vi "Single Channel Strain Configure 4Wire.vi"(5 "Channel":string, 6 "SampTime":dbl, 7 "SampCount":i32 format="%.0g", 8 "error in (no error)":errorcluster {"code" format="%.0x"}, 9 "GaugeFactor":dbl, 10 "GaugeResistance":dbl, 11 "instrument handle":refnum<k15>) -> (0 "error out":errorcluster {"code" format="%.0x"}, 3 "instrument handle out":refnum<k15>)   [LabVIEW 2020, in "Keysight DAQ970.lvlib"]
doc: "Configures a single channel for direct 4-wire strain gauge DMM digitizing, but they do not initiate the digitizing. This command redefines the scan list."
uses:
  Keysight DAQ970.lvlib
  KtDAQ970.dll
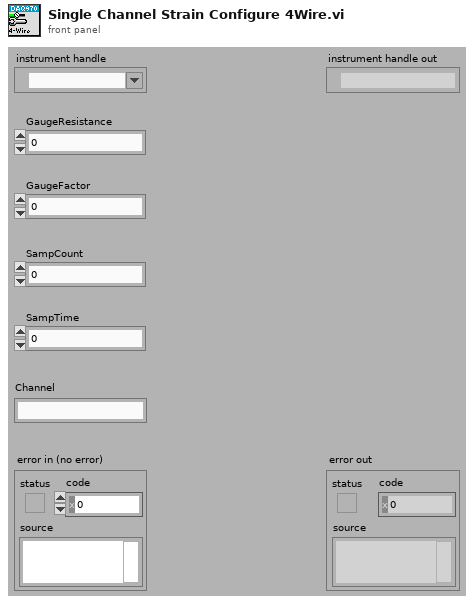
[diagram p1: front panel]
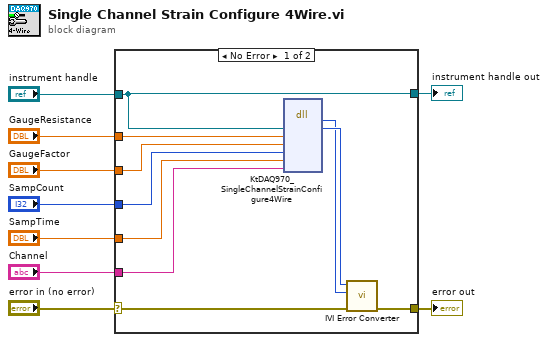
[diagram p0: block diagram]
diagram:
  n1 = case shown="No Error" "error in (no error)" {
    selector: "error in (no error)" -> [w10 w21]
    tunnel: [w17 w21] -> w9
    tunnel: "instrument handle" -> [w11 w20]
    tunnel: "GaugeResistance" -> [w16 _]
    tunnel: "GaugeFactor" -> [w15 _]
    tunnel: "SampCount" -> [w14 _]
    tunnel: "SampTime" -> [w13 _]
    tunnel: "Channel" -> [w12 _]
    tunnel: [w11 w20] -> w1
    frame No Error {
      n2 = dll-call lib="KtDAQ970**.dll" fn="KtDAQ970_SingleChannelStrainConfigure4Wire"("Vi"=w11, "GaugeResistance"=w16, "GaugeFactor"=w15, "SampCount"=w14, "SampTime"=w13, "Channel"=w12) -> (w18:i32, "Vi"=w19:u32)  [unwired: 8 in, 2 out]
      n3 = call "IVI Error Converter.vi"("error in (no error)"=w10, "IVI error code (0)"=w18, "instrument handle"=w19) -> ("error out"=w17:errorcluster)  [unwired: 7 in, 1 out]
    }
    frame Error {
    }
  }
  "error out" <- w9
  "instrument handle out" <- w1
